vi "Write Text File.vi"(8 "error in (no error)":errorcluster, 10 "Data":dbl[](array[numeric]), 11 "Path":path) -> (0 "error out":errorcluster)   [LabVIEW 2020]
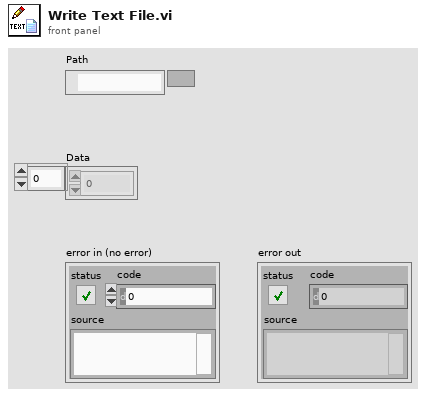
[diagram p1: front panel]
types:
  T1 = enum16{"open", "replace", "create", "open or create", "replace or create", "replace or create with confirmation"}
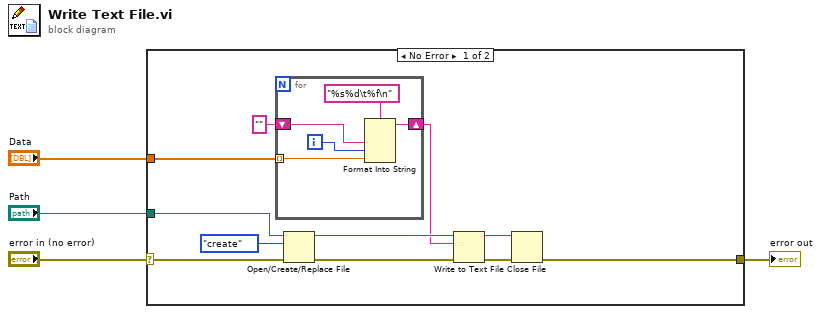
[diagram p0: block diagram]
diagram:
  n1 = case shown="No Error" "error in (no error)" {
    selector: "error in (no error)" -> [w11 w21]
    tunnel: [w9 w21] -> w3
    tunnel: "Data" -> [w7 _]
    tunnel: "Path" -> [w10 _]
    frame No Error {
      n2 = for {
        tunnel: w7 -> [w19] mode=indexing
        shift-right: [w18] -> w6
        shift-left: "" -> [w16]
        i -> [w17]
        n3 = Format Into String(format string="%s%d\t%f\n", w16, w17, w19) -> (resulting string=w18:string)  [unwired: 2 in, 1 out]
      }
      n4 = Open/Create/Replace File(file path (use dialog)=w10, error in=w11, operation (0:open)=T1."create") -> (refnum out=w15:refnum<file>, error out=w14:errorcluster)  [unwired: 3 in, 1 out]
      n5 = Write to Text File(file (use dialog)=w15, text=w6, error in=w14) -> (refnum out=w13:refnum<file>, error out=w12:errorcluster)  [unwired: 1 in, 1 out]
      n6 = Close File(refnum=w13, error in=w12) -> (error out=w9:errorcluster)  [unwired: 1 out]
    }
    frame Error {
    }
  }
  "error out" <- w3
